vi "Car Wash.vi"() -> ()   [LabVIEW 2016]
doc: "This VI allows you to simulate a car wash. The wash options controls allow you to determine which cycles will be performed. If none are selected, the High Pressure Wash cycle is the default. Once the start button is clicked, the wash begins. Use the Car Position Simulation control to simulate the position of the vehicle. If the vehicle is in the wrong position for the current cycle, the wash indicators will indicate that and you should change the car position. The Car wash display will give the current status of the wash cycle. The \"Stop Program\" button will stop the car wash immediately."
uses:
  Controls/Wash Options.ctl
  Controls/Car Position Control.ctl
  Controls/Car Wash Indicators.ctl
  Controls/State Control Enum.ctl
panel:
  in  "Stop":bool
  out "Elapsed Time":dbl format="%#.2g"
  out "Wash Indicators":T1
  in  "Car Position Slider":T2 scale=0.0..4.0
  out "Wash Entry":bool
  in  "Start":bool
  in  "Wash Options":T3
  # "Entry Console"
  # "Car Wash Display"
  # "The wash options controls allow you to determine which cycles will be performed.  \n\nIf none are selected, the High Pressure Wash cycle is the default.  \n\nOnce the start button is clicked, the wash begins."
  # "The Wash Entry LED indicates whether or not the wash in vacant or in use.\n\nThe Wash Indicator LEDs indicate the current status when the wash is in use.\n\nThe Elapsed Time indicator shows the progress for the current cycle, only if it is a timed cycle."
  # "Car Position Simulation"
  # "The Car Position Slider allows you to simulate the position of a vehicle in the wash.\nThe vehicle must be at the correct station for the each wash cycle to work.  The cycles that are completed at each station are indicated below the station number.\nIf the Vehicle Out of Position LED above is green, adjust your position to the appropriate station."
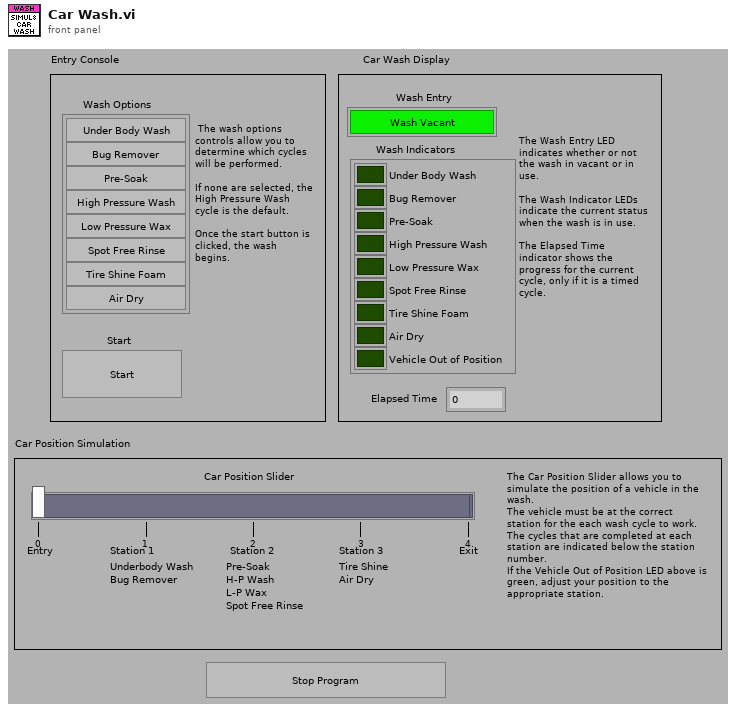
[diagram p1: front panel]
types:
  T1 = typedef "Car Wash Indicators.ctl" = cluster{"Under Body Wash":bool, "Bug Remover":bool, "Pre-Soak":bool, "High Pressure Wash":bool, "Low Pressure Wax":bool, "Spot Free Rinse":bool, "Tire Shine Foam":bool, "Air Dry":bool, "Vehicle Out of Position":bool}
  T2 = typedef "Car Position Control.ctl" = i32
  T3 = typedef "Wash Options.ctl" = cluster{"Under Body Wash":bool, "Bug Remover":bool, "Pre-Soak":bool, "High Pressure Wash":bool, "Low Pressure Wax":bool, "Spot Free Rinse":bool, "Tire Shine Foam":bool, "Air Dry":bool}
  T4 = typedef "State Control Enum.ctl" = enum16{"Initialize", "Wait for Start", "Underbody Wash", "Bug Remover", "Presoak", "HP Wash", "LP Wax", "Spot Free Rinse", "Tire Shine", "Air Dry", "Exit", "Skip", "Stop"}
  T5 = enum8{"Enabled", "Disabled", "Disabled and Grayed Out"}
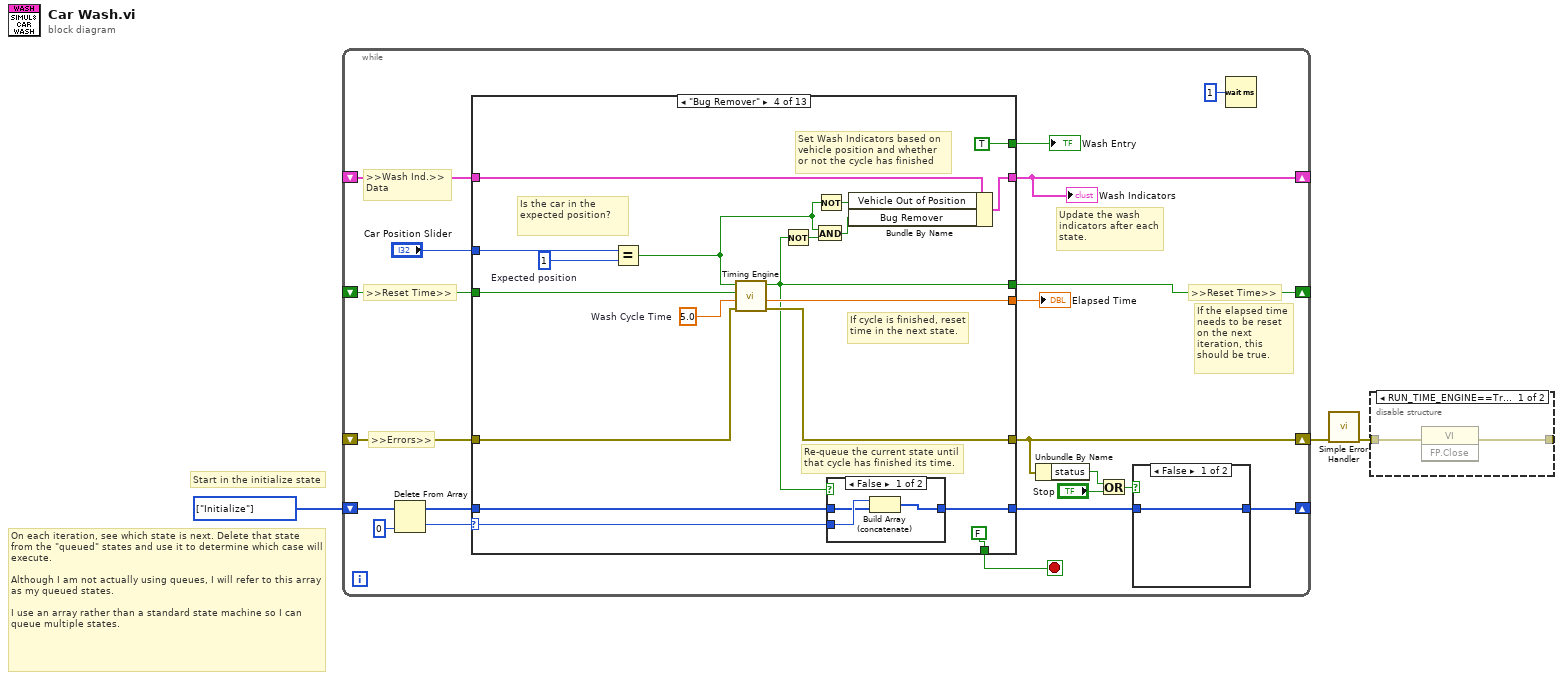
[diagram p0: block diagram]
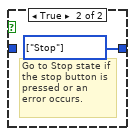
[diagram p2: hidden frame]
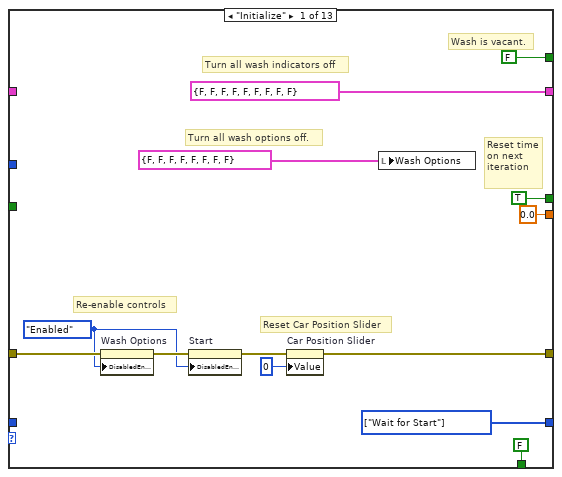
[diagram p3: hidden frame]
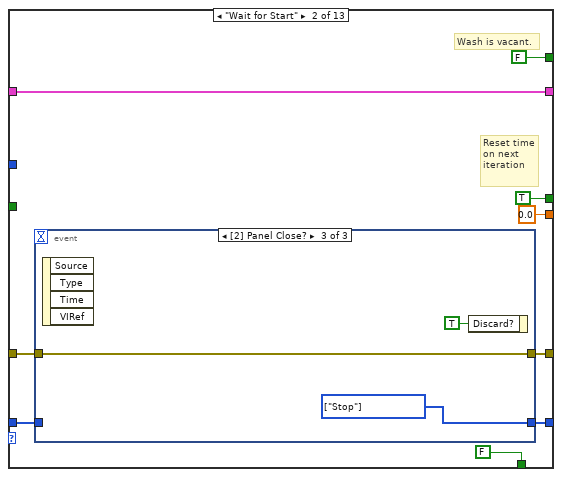
[diagram p4: hidden frame]
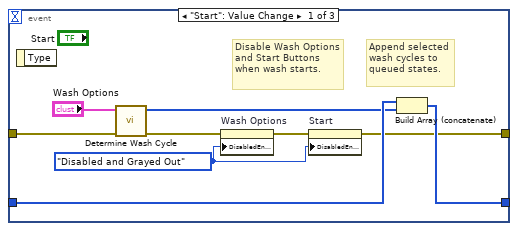
[diagram p5: hidden frame]
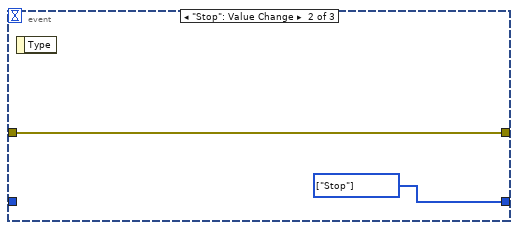
[diagram p6: hidden frame]
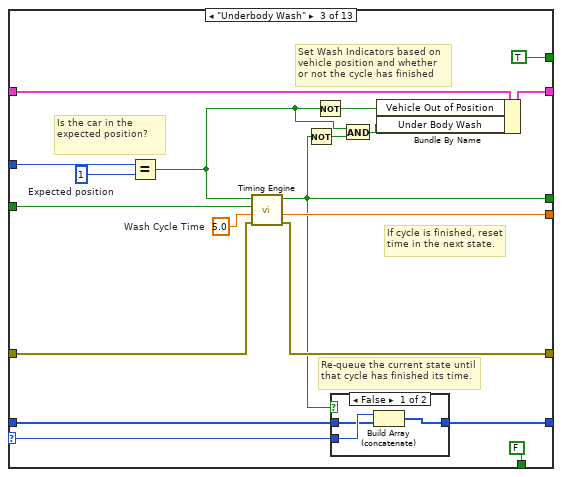
[diagram p7: hidden frame]
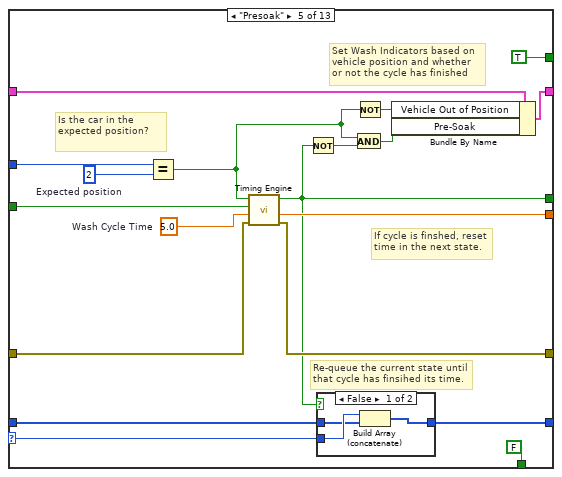
[diagram p10: hidden frame]
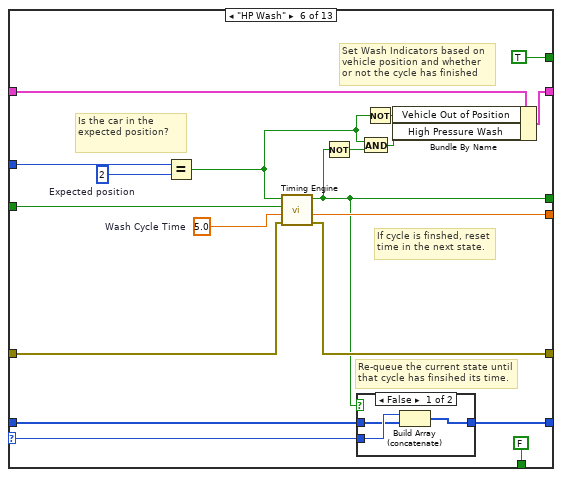
[diagram p12: hidden frame]
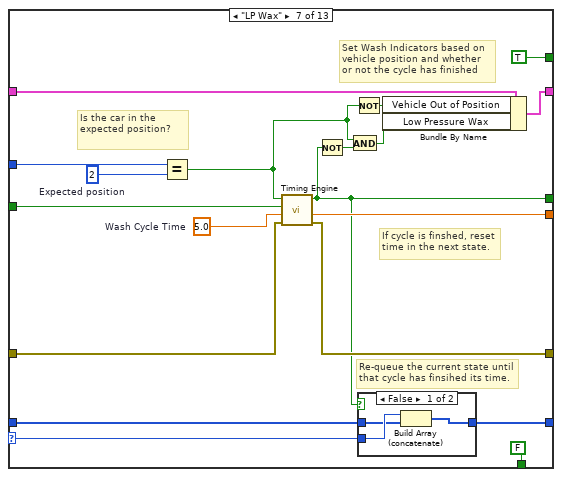
[diagram p14: hidden frame]
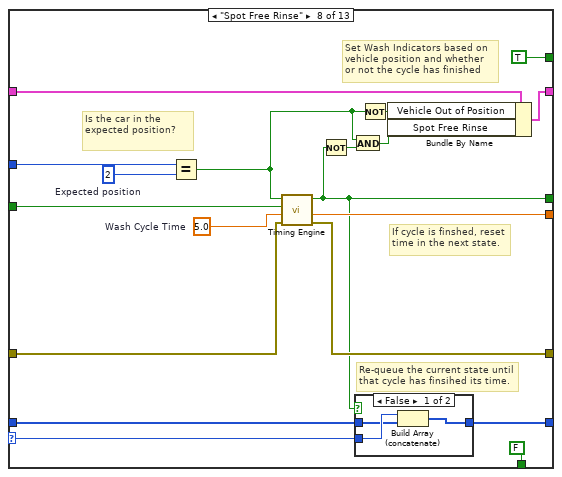
[diagram p16: hidden frame]
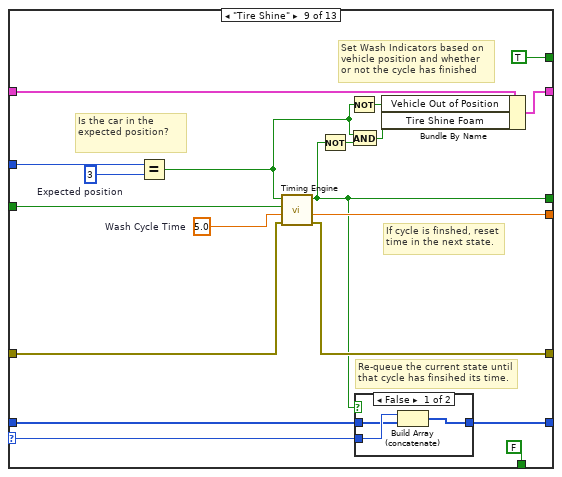
[diagram p18: hidden frame]
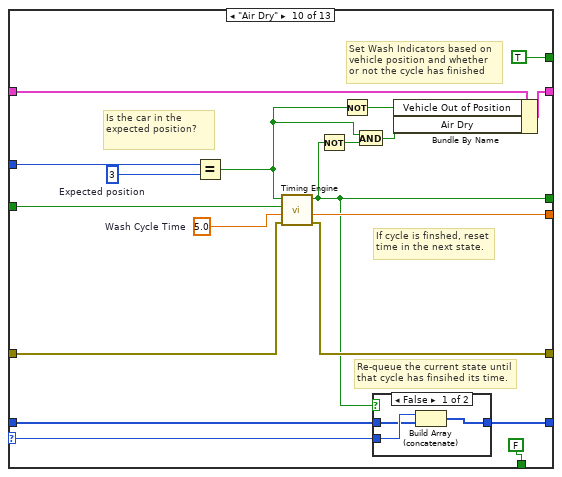
[diagram p20: hidden frame]
diagram:
  w3 = T4[] [enum."Initialize"] items=["Initialize", "Wait for Start", "Underbody Wash", "Bug Remover", "Presoak", "HP Wash", "LP Wax", "Spot Free Rinse", "Tire Shine", "Air Dry", "Exit", "Skip", "Stop"]
  # "Start in the initialize state"
  # "On each iteration, see which state is next. Delete that state from the \"queued\" states and use it to determine which case will execute. \n\nAlthough I am not actually using queues, I will refer to this array as my queued states.  \n\nI use an array rather than a standard state machine so I can queue multiple states."
  n1 = while {
    shift-right: [w15] -> _
    shift-left: w3 -> [w23]
    shift-right: [w18] -> _
    shift-left: _ -> [w19]
    shift-right: [w7] -> w2
    shift-left: _ -> [w14]
    shift-right: [w13] -> _
    shift-left: _ -> [w12]
    stop <- w9 stop-if-true
    # "Update the wash indicators after each state."
    # "If the elapsed time needs to be reset on the next iteration, this should be true."
    # ">>Reset Time>>"
    # ">>Errors>>"
    # ">>Wash Ind.>>\nData"
    # ">>Reset Time>>"
    n2 = Delete From Array(array=w23, index=0) -> (deleted portion=w20:T4, array with subset deleted=w21:T4[])  [unwired: 1 in]
    n3 = case shown="\"Bug Remover\"" w20 {
      selector: w20 -> [_ _ w69 w94 w118 w147 w163 w192 w208 w236 _ _ _]
      tunnel: w21 -> [_ w45 w68 w95 w119 w146 w162 w191 w207 w235 _ w260 _]
      tunnel: [w30 w46 w70 w93 w117 w145 w161 w184 w209 w234 w247 w260 w274] -> w16
      tunnel: [T1 {"Under Body Wash"=FALSE, "Bug Remover"=FALSE, "Pre-Soak"=FALSE, "High Pressure Wash"=FALSE, "Low Pressure Wax"=FALSE, "Spot Free Rinse"=FALSE, "Tire Shine Foam"=FALSE, "Air Dry"=FALSE, "Vehicle Out of Position"=FALSE} ("Wash Indicators 2") w39 w71 w96 w120 w139 w164 w188 w210 w237 T1 {"Under Body Wash"=FALSE, "Bug Remover"=FALSE, "Pre-Soak"=FALSE, "High Pressure Wash"=FALSE, "Low Pressure Wax"=FALSE, "Spot Free Rinse"=FALSE, "Tire Shine Foam"=FALSE, "Air Dry"=FALSE, "Vehicle Out of Position"=FALSE} ("Wash Indicators 2") w257 w276] -> w18
      tunnel: w19 -> [_ w39 w72 w97 w121 w140 w165 w189 w211 w238 _ w257 w277]
      tunnel: [FALSE ("Wash Entry") FALSE ("Wash Entry") TRUE ("Wash Entry") TRUE ("Wash Entry") TRUE ("Wash Entry") TRUE ("Wash Entry") TRUE ("Wash Entry") TRUE ("Wash Entry") TRUE ("Wash Entry") TRUE ("Wash Entry") FALSE ("Wash Entry") TRUE ("Wash Entry") TRUE ("Wash Entry")] -> w17
      tunnel: w14 -> [w36 w44 w76 w99 w113 w143 w169 w185 w216 w232 w254 w261 w270]
      tunnel: [w26 w43 w77 w98 w114 w144 w168 w193 w215 w233 w253 w262 w270] -> w7
      tunnel: [TRUE ("Time Expired?") TRUE ("Wash Entry") w62 w88 w109 w132 w157 w180 w204 w225 TRUE ("Time Expired?") w264 TRUE ("Time Expired?")] -> w13
      tunnel: w12 -> [_ _ w79 w100 w123 w142 w166 w186 w214 w231 _ w264 _]
      tunnel: [0.0 ("Elapsed Time") 0.0 ("Elapsed Time") w78 w90 w122 w138 w170 w190 w212 w239 0.0 ("Elapsed Time") w266 0.0 ("Elapsed Time")] -> w11
      tunnel: "Car Position Slider" -> [_ _ w74 w101 w124 w141 w167 w187 w213 w230 _ _ w268]
      tunnel: [FALSE ("Wash Entry") FALSE ("Wash Entry") FALSE ("Wash Entry") FALSE ("Wash Entry") FALSE ("Wash Entry") FALSE ("Wash Entry") FALSE ("Wash Entry") FALSE ("Wash Entry") FALSE ("Wash Entry") FALSE ("Wash Entry") TRUE ("Wash Entry") FALSE ("Wash Entry") FALSE ("Wash Entry")] -> w9
      frame "Initialize" {
        w30 = T4[] [enum."Wait for Start"] items=["Initialize", "Wait for Start", "Underbody Wash", "Bug Remover", "Presoak", "HP Wash", "LP Wax", "Spot Free Rinse", "Tire Shine", "Air Dry", "Exit", "Skip", "Stop"]
        w27 = T5."Enabled" ("Disabled")
        # "Reset time on next iteration"
        # "Re-enable controls"
        # "Reset Car Position Slider"
        # "Wash is vacant."
        # "Turn all wash indicators off"
        # "Turn all wash options off."
        n4 = property on="Wash Options" class="Clust (strict)"(error in=w36, "DisabledEnum"=w27) -> (error out=w35:errorcluster)  [unwired: 1 in, 1 out]
        n5 = property on="Start" class="Bool"(error in=w35, "DisabledEnum"=w27) -> (error out=w29:errorcluster)  [unwired: 1 in, 1 out]
        n6 = property on="Car Position Slider" class="Slide (strict)"(error in=w29, "Value"=0) -> (error out=w26:errorcluster)  [unwired: 1 in, 1 out]
        n7 = local write "Wash Options"(T3 {"Under Body Wash"=FALSE, "Bug Remover"=FALSE, "Pre-Soak"=FALSE, "High Pressure Wash"=FALSE, "Low Pressure Wax"=FALSE, "Spot Free Rinse"=FALSE, "Tire Shine Foam"=FALSE, "Air Dry"=FALSE} ("Wash Options")) -> ()
      }
      frame "Wait for Start" {
        # "Wash is vacant."
        # "Reset time on next iteration"
        n8 = event shown="[2] Panel Close?" {
          selector: _ -> [_ _ _]
          dyn-events: _ -> [_ _ _]
          timeout: _ -> [_ _ _]
          tunnel: [w52 w58 w61] -> w46
          tunnel: w45 -> [w54 _ _]
          tunnel: [w48 w57 w60] -> w43
          tunnel: w44 -> [w49 w57 w60]
          event "Start": Value Change {
            w50 = T5."Disabled and Grayed Out" ("Disabled")
            # "Append selected wash cycles to queued states."
            # "Disable Wash Options and Start Buttons when wash starts."
            n9 = event-data() -> ()  [unwired: 1 in, 1 out]
            n10 = call "Determine Wash Cycle.vi"("error in"=w49, "Wash Options"="Wash Options") -> ("error out"=w55:errorcluster, "Wash Cycles"=w53:T4[])  [unwired: 8 in]
            n11 = property on="Wash Options" class="Clust (strict)"(error in=w55, "DisabledEnum"=w50) -> (error out=w51:errorcluster)  [unwired: 1 in, 1 out]
            n12 = property on="Start" class="Bool"(error in=w51, "DisabledEnum"=w50) -> (error out=w48:errorcluster)  [unwired: 1 in, 1 out]
            n13 = Build Array (concatenate)(w54, w53) -> (w52:T4[])
          }
          event "Stop": Value Change {
            w58 = T4[] [enum."Stop"] items=["Initialize", "Wait for Start", "Underbody Wash", "Bug Remover", "Presoak", "HP Wash", "LP Wax", "Spot Free Rinse", "Tire Shine", "Air Dry", "Exit", "Skip", "Stop"]
            n14 = event-data() -> ()  [unwired: 1 in, 1 out]
          }
          event Panel Close? {
            w61 = T4[] [enum."Stop"] items=["Initialize", "Wait for Start", "Underbody Wash", "Bug Remover", "Presoak", "HP Wash", "LP Wax", "Spot Free Rinse", "Tire Shine", "Air Dry", "Exit", "Skip", "Stop"]
            n15 = event-data() -> ()  [unwired: 1 in, 4 out]
            n16 = event-data("Discard?"=TRUE) -> ()  [unwired: 1 in, 1 out]
          }
        }
      }
      frame "Underbody Wash" {
        w73 = T2 1  # Expected position
        w75 = 5.0  # Wash Cycle Time
        # "Is the car in the expected position?"
        # "Re-queue the current state until that cycle has finished its time."
        # "If cycle is finished, reset time in the next state."
        # "Set Wash Indicators based on vehicle position and whether or not the cycle has finished"
        n17 = Equal?(x=w74, y=w73) -> (x = y?=w64:bool)
        n18 = call "Timing Engine.vi"("error in"=w76, "Time Limit"=w75, "Reset"=w79, "Advance Time?"=w64) -> ("error out"=w77:errorcluster, "Elapsed Time"=w78:dbl, "Time Expired?"=w62:bool)  [unwired: 5 in]
        n19 = Not(x=w62) -> (.not. x?=w65:bool)
        n20 = Not(x=w64) -> (.not. x?=w67:bool)
        n21 = case shown="False" w62 {
          tunnel: [w83 w84] -> w70
          tunnel: w69 -> [w82 _]
          tunnel: w68 -> [w81 w84]
          frame False {
            n22 = Build Array (concatenate)(w82, w81) -> (w83:T4[])
          }
          frame True {
          }
        }
        n23 = And(x=w64, y=w65) -> (x .and. y?=w63:bool)
        n24 = Bundle By Name(cluster=w72, "Vehicle Out of Position"=w67, "Under Body Wash"=w63) -> (w71:T1)
      }
      frame "Bug Remover" {
        w85 = T2 1  # Expected position
        w102 = 5.0  # Wash Cycle Time
        # "Is the car in the expected position?"
        # "Re-queue the current state until that cycle has finished its time."
        # "If cycle is finished, reset time in the next state."
        # "Set Wash Indicators based on vehicle position and whether or not the cycle has finished"
        n25 = Equal?(x=w101, y=w85) -> (x = y?=w87:bool)
        n26 = call "Timing Engine.vi"("error in"=w99, "Time Limit"=w102, "Reset"=w100, "Advance Time?"=w87) -> ("error out"=w98:errorcluster, "Elapsed Time"=w90:dbl, "Time Expired?"=w88:bool)  [unwired: 5 in]
        n27 = Not(x=w88) -> (.not. x?=w89:bool)
        n28 = And(x=w87, y=w89) -> (x .and. y?=w86:bool)
        n29 = Not(x=w87) -> (.not. x?=w92:bool)
        n30 = case shown="False" w88 {
          tunnel: [w106 w107] -> w93
          tunnel: w94 -> [w105 _]
          tunnel: w95 -> [w104 w107]
          frame False {
            n31 = Build Array (concatenate)(w105, w104) -> (w106:T4[])
          }
          frame True {
          }
        }
        n32 = Bundle By Name(cluster=w97, "Vehicle Out of Position"=w92, "Bug Remover"=w86) -> (w96:T1)
      }
      frame "Presoak" {
        w108 = T2 2  # Expected position
        w125 = 5.0  # Wash Cycle Time
        # "Is the car in the expected position?"
        # "Re-queue the current state until that cycle has finsihed its time."
        # "If cycle is finshed, reset time in the next state."
        # "Set Wash Indicators based on vehicle position and whether or not the cycle has finished"
        n33 = Equal?(x=w124, y=w108) -> (x = y?=w111:bool)
        n34 = call "Timing Engine.vi"("error in"=w113, "Time Limit"=w125, "Reset"=w123, "Advance Time?"=w111) -> ("error out"=w114:errorcluster, "Elapsed Time"=w122:dbl, "Time Expired?"=w109:bool)  [unwired: 5 in]
        n35 = Not(x=w109) -> (.not. x?=w112:bool)
        n36 = case shown="False" w109 {
          tunnel: [w129 w130] -> w117
          tunnel: w118 -> [w128 _]
          tunnel: w119 -> [w127 w130]
          frame False {
            n37 = Build Array (concatenate)(w128, w127) -> (w129:T4[])
          }
          frame True {
          }
        }
        n38 = And(x=w111, y=w112) -> (x .and. y?=w110:bool)
        n39 = Not(x=w111) -> (.not. x?=w116:bool)
        n40 = Bundle By Name(cluster=w121, "Vehicle Out of Position"=w116, "Pre-Soak"=w110) -> (w120:T1)
      }
      frame "HP Wash" {
        w131 = T2 2  # Expected position
        w148 = 5.0  # Wash Cycle Time
        # "Is the car in the expected position?"
        # "Re-queue the current state until that cycle has finsihed its time."
        # "If cycle is finshed, reset time in the next state."
        # "Set Wash Indicators based on vehicle position and whether or not the cycle has finished"
        n41 = Equal?(x=w141, y=w131) -> (x = y?=w133:bool)
        n42 = call "Timing Engine.vi"("error in"=w143, "Time Limit"=w148, "Reset"=w142, "Advance Time?"=w133) -> ("error out"=w144:errorcluster, "Elapsed Time"=w138:dbl, "Time Expired?"=w132:bool)  [unwired: 5 in]
        n43 = Not(x=w132) -> (.not. x?=w135:bool)
        n44 = case shown="False" w132 {
          tunnel: [w152 w153] -> w145
          tunnel: w147 -> [w151 _]
          tunnel: w146 -> [w150 w153]
          frame False {
            n45 = Build Array (concatenate)(w151, w150) -> (w152:T4[])
          }
          frame True {
          }
        }
        n46 = And(x=w133, y=w135) -> (x .and. y?=w134:bool)
        n47 = Not(x=w133) -> (.not. x?=w137:bool)
        n48 = Bundle By Name(cluster=w140, "Vehicle Out of Position"=w137, "High Pressure Wash"=w134) -> (w139:T1)
      }
      frame "LP Wax" {
        w154 = T2 2  # Expected position
        w171 = 5.0  # Wash Cycle Time
        # "Is the car in the expected position?"
        # "Re-queue the current state until that cycle has finsihed its time."
        # "If cycle is finshed, reset time in the next state."
        # "Set Wash Indicators based on vehicle position and whether or not the cycle has finished"
        n49 = Equal?(x=w167, y=w154) -> (x = y?=w156:bool)
        n50 = call "Timing Engine.vi"("error in"=w169, "Time Limit"=w171, "Reset"=w166, "Advance Time?"=w156) -> ("error out"=w168:errorcluster, "Elapsed Time"=w170:dbl, "Time Expired?"=w157:bool)  [unwired: 5 in]
        n51 = Not(x=w157) -> (.not. x?=w158:bool)
        n52 = And(x=w156, y=w158) -> (x .and. y?=w155:bool)
        n53 = Not(x=w156) -> (.not. x?=w160:bool)
        n54 = case shown="False" w157 {
          tunnel: [w175 w176] -> w161
          tunnel: w163 -> [w174 _]
          tunnel: w162 -> [w173 w176]
          frame False {
            n55 = Build Array (concatenate)(w174, w173) -> (w175:T4[])
          }
          frame True {
          }
        }
        n56 = Bundle By Name(cluster=w165, "Vehicle Out of Position"=w160, "Low Pressure Wax"=w155) -> (w164:T1)
      }
      frame "Spot Free Rinse" {
        w177 = T2 2  # Expected position
        w194 = 5.0  # Wash Cycle Time
        # "Is the car in the expected position?"
        # "Re-queue the current state until that cycle has finsihed its time."
        # "If cycle is finshed, reset time in the next state."
        # "Set Wash Indicators based on vehicle position and whether or not the cycle has finished"
        n57 = Equal?(x=w187, y=w177) -> (x = y?=w179:bool)
        n58 = call "Timing Engine.vi"("error in"=w185, "Time Limit"=w194, "Reset"=w186, "Advance Time?"=w179) -> ("error out"=w193:errorcluster, "Elapsed Time"=w190:dbl, "Time Expired?"=w180:bool)  [unwired: 5 in]
        n59 = Not(x=w180) -> (.not. x?=w181:bool)
        n60 = And(x=w179, y=w181) -> (x .and. y?=w178:bool)
        n61 = case shown="False" w180 {
          tunnel: [w198 w199] -> w184
          tunnel: w192 -> [w197 _]
          tunnel: w191 -> [w196 w199]
          frame False {
            n62 = Build Array (concatenate)(w197, w196) -> (w198:T4[])
          }
          frame True {
          }
        }
        n63 = Not(x=w179) -> (.not. x?=w183:bool)
        n64 = Bundle By Name(cluster=w189, "Vehicle Out of Position"=w183, "Spot Free Rinse"=w178) -> (w188:T1)
      }
      frame "Tire Shine" {
        w200 = T2 3  # Expected position
        w217 = 5.0  # Wash Cycle Time
        # "Is the car in the expected position?"
        # "Re-queue the current state until that cycle has finsihed its time."
        # "If cycle is finshed, reset time in the next state."
        # "Set Wash Indicators based on vehicle position and whether or not the cycle has finished"
        n65 = Equal?(x=w213, y=w200) -> (x = y?=w202:bool)
        n66 = call "Timing Engine.vi"("error in"=w216, "Time Limit"=w217, "Reset"=w214, "Advance Time?"=w202) -> ("error out"=w215:errorcluster, "Elapsed Time"=w212:dbl, "Time Expired?"=w204:bool)  [unwired: 5 in]
        n67 = Not(x=w204) -> (.not. x?=w203:bool)
        n68 = Not(x=w202) -> (.not. x?=w206:bool)
        n69 = And(x=w202, y=w203) -> (x .and. y?=w201:bool)
        n70 = case shown="False" w204 {
          tunnel: [w221 w222] -> w209
          tunnel: w208 -> [w220 _]
          tunnel: w207 -> [w219 w222]
          frame False {
            n71 = Build Array (concatenate)(w220, w219) -> (w221:T4[])
          }
          frame True {
          }
        }
        n72 = Bundle By Name(cluster=w211, "Vehicle Out of Position"=w206, "Tire Shine Foam"=w201) -> (w210:T1)
      }
      frame "Air Dry" {
        w223 = T2 3  # Expected position
        w240 = 5.0  # Wash Cycle Time
        # "Is the car in the expected position?"
        # "If cycle is finshed, reset time in the next state."
        # "Re-queue the current state until that cycle has finsihed its time."
        # "Set Wash Indicators based on vehicle position and whether or not the cycle has finished"
        n73 = Equal?(x=w230, y=w223) -> (x = y?=w226:bool)
        n74 = call "Timing Engine.vi"("error in"=w232, "Time Limit"=w240, "Reset"=w231, "Advance Time?"=w226) -> ("error out"=w233:errorcluster, "Elapsed Time"=w239:dbl, "Time Expired?"=w225:bool)  [unwired: 5 in]
        n75 = Not(x=w225) -> (.not. x?=w227:bool)
        n76 = Not(x=w226) -> (.not. x?=w229:bool)
        n77 = And(x=w226, y=w227) -> (x .and. y?=w224:bool)
        n78 = case shown="False" w225 {
          tunnel: [w244 w245] -> w234
          tunnel: w236 -> [w243 _]
          tunnel: w235 -> [w242 w245]
          frame False {
            n79 = Build Array (concatenate)(w243, w242) -> (w244:T4[])
          }
          frame True {
          }
        }
        n80 = Bundle By Name(cluster=w238, "Vehicle Out of Position"=w229, "Air Dry"=w224) -> (w237:T1)
      }
      frame "Stop" {
        w247 = T4[] [enum."Stop"] items=["Initialize", "Wait for Start", "Underbody Wash", "Bug Remover", "Presoak", "HP Wash", "LP Wax", "Spot Free Rinse", "Tire Shine", "Air Dry", "Exit", "Skip", "Stop"]
        w252 = T5."Enabled" ("Disabled")
        # "Reset time on next iteration"
        # "Reset the car's position to Entry"
        # "Re-enable FP controls"
        n81 = local write "Car Position Slider"(T2 0 ("Car Position Slider")) -> ()
        n82 = property on="Wash Options" class="Clust (strict)"(error in=w254, "DisabledEnum"=w252) -> (error out=w255:errorcluster)  [unwired: 1 in, 1 out]
        n83 = property on="Start" class="Bool"(error in=w255, "DisabledEnum"=w252) -> (error out=w253:errorcluster)  [unwired: 1 in, 1 out]
      }
      frame "Skip" {
        w258 = 0.0  # Time Limit
        # "In the skip state, the only action done is to call the timing VI so the timestamp is updated."
        n84 = call "Timing Engine.vi"("error in"=w261, "Time Limit"=w258, "Reset"=w264, "Advance Time?"=FALSE) -> ("error out"=w262:errorcluster, "Elapsed Time"=w266:dbl)  [unwired: 5 in, 1 out]
      }
      frame "Exit" {
        w267 = T2 4  # Expected position
        # "Is the car in the expected position?"
        # "Reset time on next iteration"
        # "Stay in the exit position until the car has moved to exit. The go to initialize state."
        n85 = Not Equal?(x=w268, y=w267) -> (x != y?=w275:bool)
        n86 = case shown="True" w275 {
          tunnel: [w278 w279] -> w274
          frame False {
            w278 = T4[] [enum."Initialize"] items=["Initialize", "Wait for Start", "Underbody Wash", "Bug Remover", "Presoak", "HP Wash", "LP Wax", "Spot Free Rinse", "Tire Shine", "Air Dry", "Exit", "Skip", "Stop"]
          }
          frame True {
            w279 = T4[] [enum."Exit"] items=["Initialize", "Wait for Start", "Underbody Wash", "Bug Remover", "Presoak", "HP Wash", "LP Wax", "Spot Free Rinse", "Tire Shine", "Air Dry", "Exit", "Skip", "Stop"]
          }
        }
        n87 = Bundle By Name(cluster=w277, "Vehicle Out of Position"=w275) -> (w276:T1)
      }
    }
    "Wash Indicators" <- w18
    "Wash Entry" <- w17
    "Elapsed Time" <- w11
    n88 = Unbundle By Name(w7) -> ("status"=w6:bool)
    n89 = Or(x=w6, y="Stop") -> (x .or. y?=w4:bool)
    n90 = case shown="False" w4 {
      tunnel: w16 -> [w24 _]
      tunnel: [w24 w25] -> w15
      frame False {
      }
      frame True {
        w25 = T4[] [enum."Stop"] items=["Initialize", "Wait for Start", "Underbody Wash", "Bug Remover", "Presoak", "HP Wash", "LP Wax", "Spot Free Rinse", "Tire Shine", "Air Dry", "Exit", "Skip", "Stop"]
        # "Go to Stop state if the stop button is pressed or an error occurs."
      }
    }
    n91 = Wait (ms)(milliseconds to wait=u32 1) -> ()  [unwired: 1 out]
  }
  n92 = call <vilib>:"Simple Error Handler.vi"("error in (no error)"=w2) -> ("error out"=w1:errorcluster)  [unwired: 4 in, 4 out]
  n93 = disable-structure shown="RUN_TIME_ENGINE==True" {
    disable-tunnel: w1 -> [w281 w282]
    disable-tunnel: [w280 w282] -> _
    frame condition #0 {
      n94 = invoke class="VI" method="FP.Close"(error in=w281) -> (error out=w280:errorcluster)  [unwired: 2 in, 2 out]
    }
    frame condition #1 (active) {
    }
  }
